vi "Open.vi"(8 "error in (no error)":errorcluster caption="entrée d'erreur (pas d'erreur)", 11 "Class Balance_Adam_GBK en entrée":refnum<class "Class Balance_Adam_GBK.lvclass">) -> (0 "error out":errorcluster caption="sortie d'erreur", 3 "Class Balance_Adam_GBK en sortie":refnum<class "Class Balance_Adam_GBK.lvclass">)   [LabVIEW 2020, in "Library Instrument & Equipement.lvlib" / "Library Balance.lvlib" / "Class Balance_Adam_GBK.lvclass"]
uses:
  Class Balance_Adam_GBK.lvclass
  C:/Users/ngarcin/OneDrive - Altyor/Standard TB/Class/Balance/Balance (Default)/Class Balance (Default).lvclass
  Class Balance_Adam_GBK.lvclass/Class Balance_Adam_GBK.ctl
  <vilib>/Instr/_visa.llb/VISA Configure Serial Port (Instr).vi
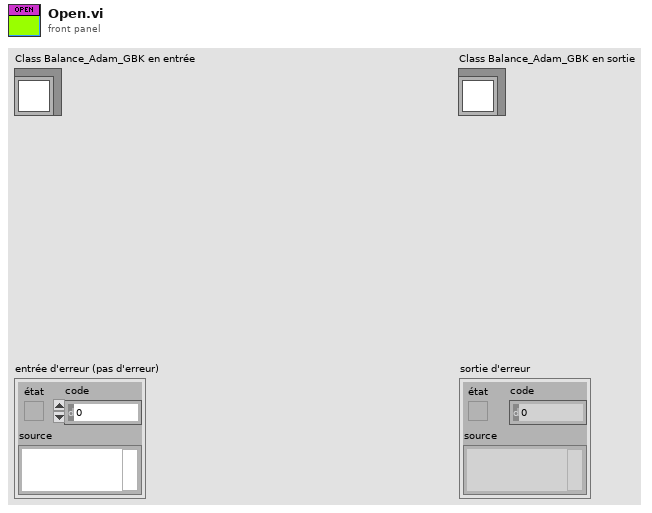
[diagram p1: front panel]
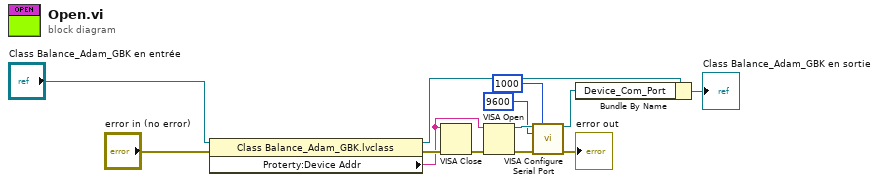
[diagram p0: block diagram]
diagram:
  n1 = property class="Class Balance_Adam_GBK.lvclass"(reference="Class Balance_Adam_GBK en entrée", error in="error in (no error)") -> (reference out=w4:refnum<class "Class Balance_Adam_GBK.lvclass">, error out=w9:errorcluster, "Proterty:Device Addr"=w8:string)
  n2 = VISA Close(VISA resource name=w8, error in (no error)=w9) -> (error out=w10:errorcluster)
  n3 = VISA Open(error in (no error)=w10, VISA resource name=w8) -> (VISA resource name=w13:refnum<visa-resource-name>, error out=w11:errorcluster)  [unwired: 3 in]
  n4 = call-poly "VISA Configure Serial Port"("VISA resource name"=w13, "timeout (10sec)"=u32 1000, "baud rate (9600)"=u32 9600, "error in (no error)"=w11) -> ("VISA resource name out"=w2:refnum<visa-resource-name>, "error out"=→"error out":errorcluster)  [unwired: 10 in]
  n5 = Bundle By Name(cluster=w4, "Device_Com_Port"=w2) -> (→"Class Balance_Adam_GBK en sortie":refnum<class "Class Balance_Adam_GBK.lvclass">)
